vi "BLE Pointer - Main.vi"() -> ()   [LabVIEW 2016]
uses:
  Typedef/SM - Pointer.ctl
  <vilib>/Analysis/coordinate.llb/Angle Units.ctl
  <vilib>/Analysis/coordinate.llb/Absolute Angle Difference (scalar).vi
  <vilib>/Analysis/coordinate.llb/Wrap Angle (scalar).vi
  <vilib>/Analysis/coordinate.llb/Set Angle Unit.vi
  User32.dll
  <vilib>/Analysis/NI_AAL_Angle.lvlib
panel:
  out "YPR data":cluster{"Yaw":sgl, "Pitch":sgl, "Roll":sgl}
  out "Roll range":dbl
  out "Yaw range":dbl
  out "BR Point":cluster{"BR Yaw":sgl, "BR Roll":sgl}
  out "TL Point":cluster{"TL Yaw":sgl, "TL Roll":sgl}
  out "Y":i32
  out "X":i32
  in  "Track":bool
  in  "Set Bottom right":bool
  in  "Exit":bool
  in  "Set Left up":bool
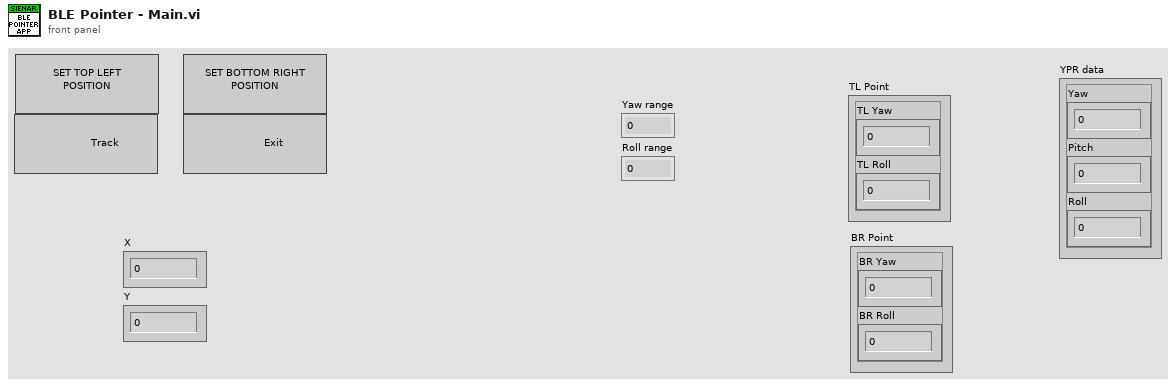
[diagram p1: front panel]
types:
  T1 = cluster{"Strain data":cluster{"Strain sensor 1":sgl, "Strain sensor 2":sgl, "Strain sensor 3":sgl, "Strain sensor 4":sgl, "Strain sensor 5":sgl, "Strain sensor 6":sgl, "Strain sensor 7":sgl, "Strain sensor 8":sgl}, "YPR data":cluster{"Yaw":sgl, "Pitch":sgl, "Roll":sgl}}
  T2 = cluster{"BR Point":cluster{"BR Yaw":sgl, "BR Roll":sgl}, "TL Point":cluster{"TL Yaw":sgl, "TL Roll":sgl}}
  T3 = typedef "SM - Pointer.ctl" = enum16{"Set Top left corner", "Set Bottom right corner", "Stop", "Track", "Exit"}
  T4 = typedef "NI_AAL_Angle.lvlib/Angle Units.ctl" = i32
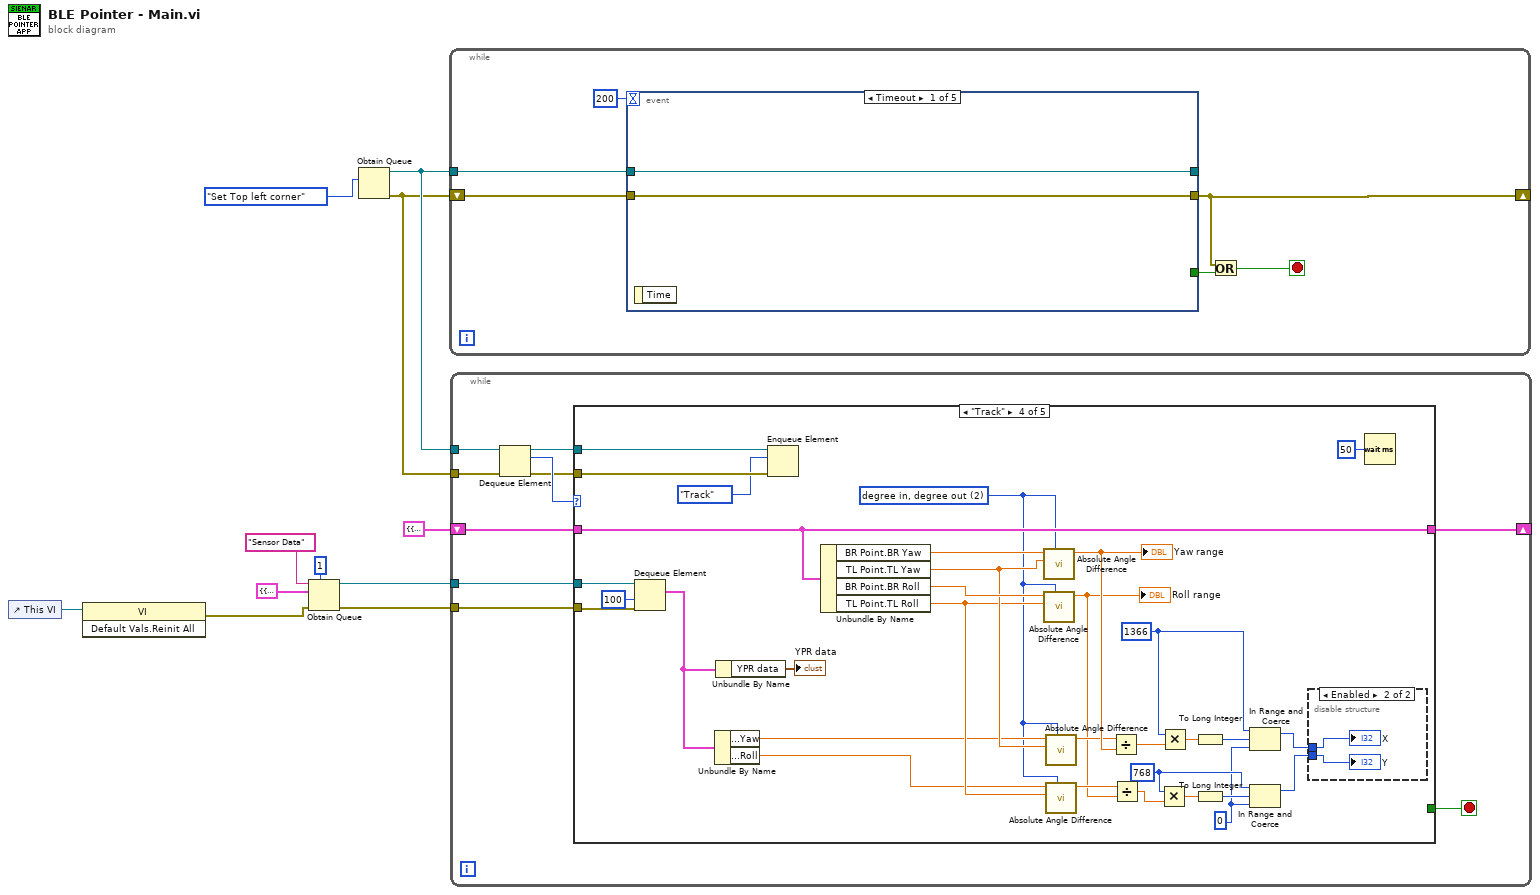
[diagram p0: block diagram]
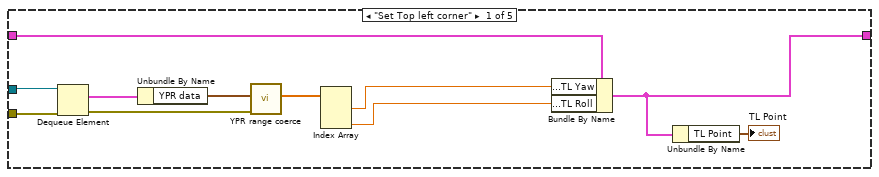
[diagram p2: hidden frame]
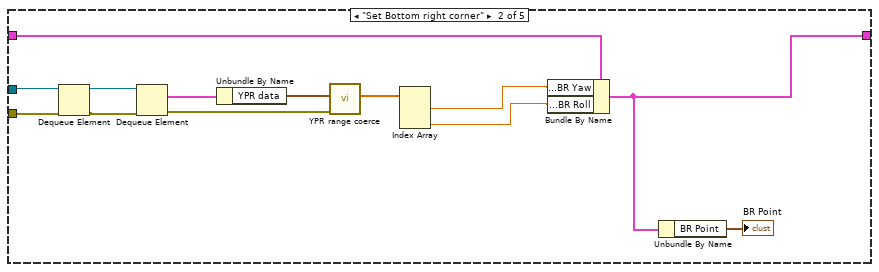
[diagram p3: hidden frame]
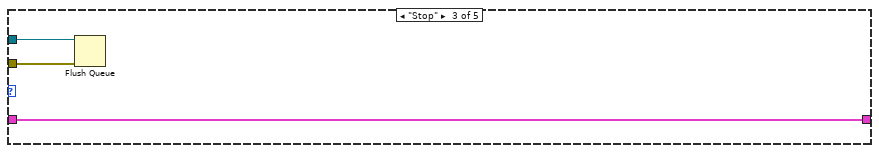
[diagram p4: hidden frame]
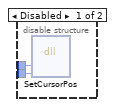
[diagram p5: hidden frame]
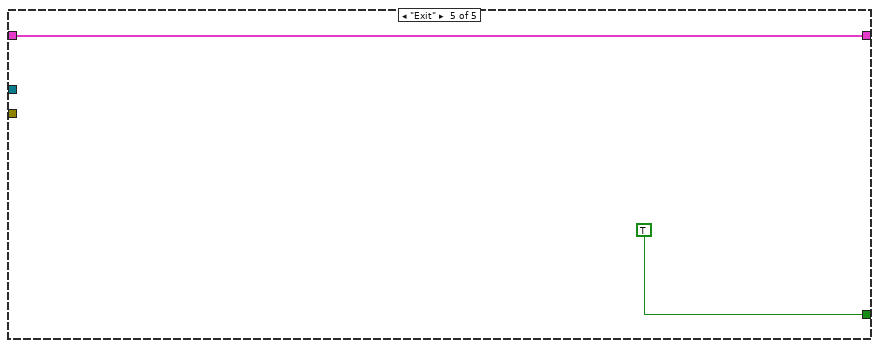
[diagram p6: hidden frame]
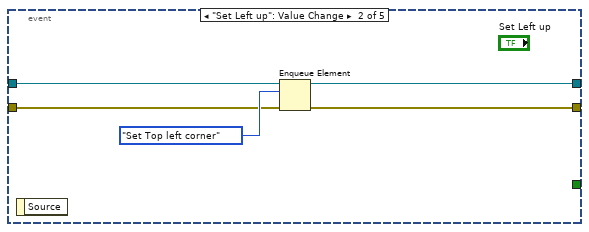
[diagram p7: hidden frame]
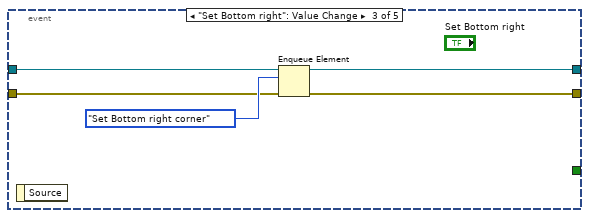
[diagram p8: hidden frame]
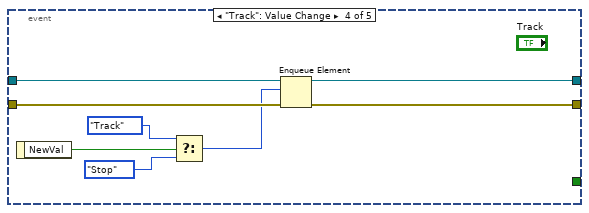
[diagram p9: hidden frame]
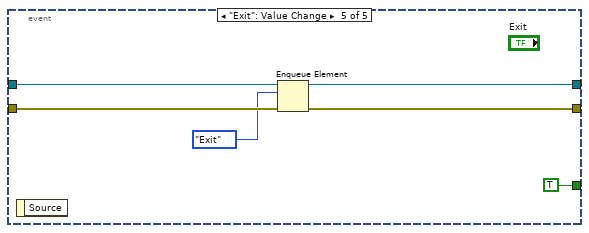
[diagram p10: hidden frame]
diagram:
  n1 = control-ref of="This VI"() -> (w2:refnum<vi>)
  n2 = invoke class="VI" method="Default Vals.Reinit All"(reference=w2) -> (error out=w1:errorcluster)  [unwired: 2 in, 2 out]
  n3 = Obtain Queue(max queue size (-1, unlimited)=1, name (unnamed)="Sensor Data", element data type=T1 {"Strain data"={"Strain sensor 1"=0.0, "Strain sensor 2"=0.0, "Strain sensor 3"=0.0, "Strain sensor 4"=0.0, "Strain sensor 5"=0.0, "Strain sensor 6"=0.0, "Strain sensor 7"=0.0, "Strain sensor 8"=0.0}, "YPR data"={"Yaw"=0.0, "Pitch"=0.0, "Roll"=0.0}} ("Wristband data"), error in (no error)=w1) -> (queue out=w4:refnum<queue>, error out=w3:errorcluster)  [unwired: 1 in, 1 out]
  n4 = Obtain Queue(element data type=SM_-_Pointer."Set Top left corner") -> (queue out=w10:refnum<queue>, error out=w9:errorcluster)  [unwired: 4 in, 1 out]
  n5 = while {
    tunnel: w10 -> [w17]
    shift-right: [w13] -> _
    shift-left: w9 -> [w16]
    stop <- w12 stop-if-true
    n6 = event shown="[0] Timeout" {
      selector: _ -> [_ _ _ _ _]
      dyn-events: _ -> [_ _ _ _ _]
      timeout: 200 -> [_ _ _ _ _]
      tunnel: w17 -> [w19 w23 w28 w37 w43]
      tunnel: w16 -> [w18 w22 w27 w36 w42]
      tunnel: [w19 w20 w25 w34 w41] -> _
      tunnel: [w18 w21 w26 w35 w40] -> w13
      tunnel: [_ _ _ _ TRUE] -> w14
      event Timeout {
        n7 = event-data() -> ()  [unwired: 1 in, 1 out]
      }
      event "Set Left up": Value Change {
        n8 = event-data() -> ()  [unwired: 1 in, 1 out]
        n9 = Enqueue Element(queue=w23, element=SM_-_Pointer."Set Top left corner", error in (no error)=w22) -> (queue out=w20:refnum<queue>, error out=w21:errorcluster)  [unwired: 1 in, 1 out]
      }
      event "Set Bottom right": Value Change {
        n10 = event-data() -> ()  [unwired: 1 in, 1 out]
        n11 = Enqueue Element(queue=w28, element=SM_-_Pointer."Set Bottom right corner", error in (no error)=w27) -> (queue out=w25:refnum<queue>, error out=w26:errorcluster)  [unwired: 1 in, 1 out]
      }
      event "Track": Value Change {
        n12 = event-data() -> ("NewVal"=w33:bool)  [unwired: 1 in]
        n13 = Select(t=SM_-_Pointer."Track", s=w33, f=SM_-_Pointer."Stop") -> (s? t:f=w30:T3)
        n14 = Enqueue Element(queue=w37, element=w30, error in (no error)=w36) -> (queue out=w34:refnum<queue>, error out=w35:errorcluster)  [unwired: 1 in, 1 out]
      }
      event "Exit": Value Change {
        n15 = event-data() -> ()  [unwired: 1 in, 1 out]
        n16 = Enqueue Element(queue=w43, element=SM_-_Pointer."Exit", error in (no error)=w42) -> (queue out=w41:refnum<queue>, error out=w40:errorcluster)  [unwired: 1 in, 1 out]
      }
    }
    n17 = Or(x=w13, y=w14) -> (x .or. y?=w12:bool)
  }
  n18 = while {
    tunnel: w10 -> [w53]
    tunnel: w9 -> [w52]
    shift-right: [w46] -> _
    shift-left: T2 {"BR Point"={"BR Yaw"=0.0, "BR Roll"=0.0}, "TL Point"={"TL Yaw"=0.0, "TL Roll"=0.0}} -> [w49]
    tunnel: w4 -> [w48]
    tunnel: w3 -> [w47]
    stop <- w50 stop-if-true
    n19 = Dequeue Element(queue=w53, error in (no error)=w52) -> (queue out=w45:refnum<queue>, element=w51:T3, error out=w44:errorcluster)  [unwired: 1 in, 1 out]
    n20 = case shown="\"Track\"" w51 {
      tunnel: [_ _ _ _ TRUE] -> w50
      tunnel: w49 -> [w62 w67 w80 w109 w117]
      tunnel: w48 -> [w64 w76 _ w111 _]
      tunnel: w47 -> [w63 w77 _ w110 _]
      tunnel: [w55 w66 w80 w109 w117] -> w46
      tunnel: w45 -> [_ _ w78 w108 _]
      tunnel: w44 -> [_ _ w79 w107 _]
      frame "Set Top left corner" {
        n21 = Dequeue Element(queue=w64, error in (no error)=w63) -> (element=w61:T1, error out=w59:errorcluster)  [unwired: 1 in, 2 out]
        n22 = Unbundle By Name(w61) -> ("YPR data"=w60:cluster{"Yaw":sgl, "Pitch":sgl, "Roll":sgl})
        n23 = call "YPR range coerce.vi"("Error In"=w59, "YPR data"=w60) -> ("YPR Array"=w58:sgl[])  [unwired: 8 in, 1 out]
        n24 = Index Array(array=w58) -> (element #1=w57:sgl, element #3=w56:sgl)  [unwired: 3 in, 1 out]
        n25 = Bundle By Name(cluster=w62, "TL Point.TL Yaw"=w57, "TL Point.TL Roll"=w56) -> (w55:T2)
        n26 = Unbundle By Name(w55) -> ("TL Point"=→"TL Point":cluster{"TL Yaw":sgl, "TL Roll":sgl})
      }
      frame "Set Bottom right corner" {
        n27 = Dequeue Element(queue=w76, error in (no error)=w77) -> (queue out=w71:refnum<queue>, error out=w70:errorcluster)  [unwired: 1 in, 2 out]
        n28 = Dequeue Element(queue=w71, error in (no error)=w70) -> (element=w75:T1, error out=w73:errorcluster)  [unwired: 1 in, 2 out]
        n29 = Unbundle By Name(w75) -> ("YPR data"=w74:cluster{"Yaw":sgl, "Pitch":sgl, "Roll":sgl})
        n30 = call "YPR range coerce.vi"("Error In"=w73, "YPR data"=w74) -> ("YPR Array"=w72:sgl[])  [unwired: 8 in, 1 out]
        n31 = Index Array(array=w72) -> (element #1=w69:sgl, element #3=w68:sgl)  [unwired: 3 in, 1 out]
        n32 = Bundle By Name(cluster=w67, "BR Point.BR Yaw"=w69, "BR Point.BR Roll"=w68) -> (w66:T2)
        n33 = Unbundle By Name(w66) -> ("BR Point"=→"BR Point":cluster{"BR Yaw":sgl, "BR Roll":sgl})
      }
      frame "Stop" {
        n34 = Flush Queue(queue=w78, error in (no error)=w79) -> ()  [unwired: 3 out]
      }
      frame "Track" {
        w84 = T4 2 items=["radian in, radian out", "radian in, degree out", "degree in, degree out", "degree in, radian out"] ("angle units")
        w97 = 0
        w104 = 1366
        w102 = 768
        n35 = Dequeue Element(queue=w111, timeout in ms (-1)=100, error in (no error)=w110) -> (element=w82:T1)  [unwired: 3 out]
        n36 = Unbundle By Name(w82) -> ("YPR data.Yaw"=w86:sgl, "YPR data.Roll"=w85:sgl)
        n37 = Unbundle By Name(w82) -> ("YPR data"=→"YPR data":cluster{"Yaw":sgl, "Pitch":sgl, "Roll":sgl})
        n38 = Enqueue Element(queue=w108, element=SM_-_Pointer."Track", error in (no error)=w107) -> ()  [unwired: 1 in, 3 out]
        n39 = Unbundle By Name(w109) -> ("BR Point.BR Yaw"=w93:sgl, "TL Point.TL Yaw"=w89:sgl, "BR Point.BR Roll"=w91:sgl, "TL Point.TL Roll"=w87:sgl)
        n40 = call-poly <vilib>:"Absolute Angle Difference.vi"("angle units"=w84, "angle 2"=w89, "angle 1"=w93) -> ("absolute angle difference"=w92:dbl)  [unwired: 7 in, 1 out]
        "Yaw range" <- w92
        n41 = call-poly <vilib>:"Absolute Angle Difference.vi"("angle units"=w84, "angle 2"=w87, "angle 1"=w91) -> ("absolute angle difference"=w83:dbl)  [unwired: 7 in, 1 out]
        "Roll range" <- w83
        n42 = call-poly <vilib>:"Absolute Angle Difference.vi"("angle units"=w84, "angle 2"=w89, "angle 1"=w86) -> ("absolute angle difference"=w90:dbl)  [unwired: 7 in, 1 out]
        n43 = call-poly <vilib>:"Absolute Angle Difference.vi"("angle units"=w84, "angle 2"=w87, "angle 1"=w85) -> ("absolute angle difference"=w88:dbl)  [unwired: 7 in, 1 out]
        n44 = Divide(x=w90, y=w92) -> (x/y=w105:dbl)
        n45 = Divide(x=w88, y=w83) -> (x/y=w103:dbl)
        n46 = Multiply(x=w102, y=w103) -> (x*y=w99:dbl)
        n47 = Multiply(x=w104, y=w105) -> (x*y=w101:dbl)
        n48 = To Long Integer(number=w101) -> (32bit integer=w100:i32)
        n49 = To Long Integer(number=w99) -> (32bit integer=w98:i32)
        n50 = In Range and Coerce(upper limit=w104, x=w100, lower limit=w97) -> (coerced(x)=w96:i32)  [unwired: 1 out]
        n51 = In Range and Coerce(upper limit=w102, x=w98, lower limit=w97) -> (coerced(x)=w95:i32)  [unwired: 1 out]
        n52 = disable-structure shown="Enabled" {
          disable-tunnel: w96 -> [w114 w116]
          disable-tunnel: w95 -> [w113 w115]
          frame Disabled {
            n53 = dll-call lib="user32.dll" fn="SetCursorPos"("dx"=w114, "dy"=w113) -> ()  [unwired: 6 in, 2 out]
          }
          frame Enabled {
            "X" <- w116
            "Y" <- w115
          }
        }
        n54 = Wait (ms)(milliseconds to wait=u32 50) -> ()  [unwired: 1 out]
      }
      frame "Exit" {
      }
    }
  }
